vi "_vna_send_command_(RS_NT_command).vi"(3 "error in (no error)":errorcluster, 4 "Comand":string="TRIG:SOUR EXT", 5 "address":string="192.168.0.3") -> (0 "error out":errorcluster)   [LabVIEW 2013]
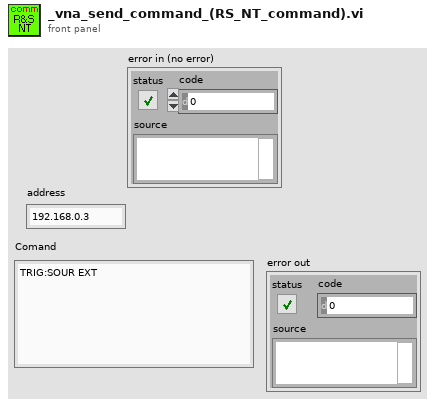
[diagram p1: front panel]
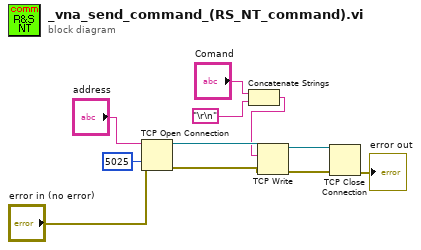
[diagram p0: block diagram]
diagram:
  n1 = TCP Open Connection(address="address", remote port or service name=u16 5025, error in (no error)="error in (no error)") -> (connection ID=w11:refnum<k5>, error out=w9:errorcluster)  [unwired: 2 in]
  n2 = Concatenate Strings("Comand", "\r\n") -> (w2:string)
  n3 = TCP Write(connection ID=w11, data in=w2, error in (no error)=w9) -> (connection ID out=w10:refnum<k5>, error out=w8:errorcluster)  [unwired: 1 in, 1 out]
  n4 = TCP Close Connection(connection ID=w10, error in (no error)=w8) -> (error out=→"error out":errorcluster)  [unwired: 1 in, 1 out]
